vi "TH_Bladmögelvarning Skylt.vi"(7 "Tid":string) -> ()   [LabVIEW 2014]
panel:
  in  "OK Button":bool
  # "Bladmögelvarning !"
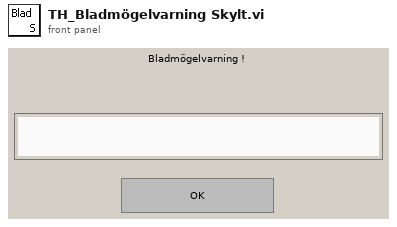
[diagram p1: front panel]
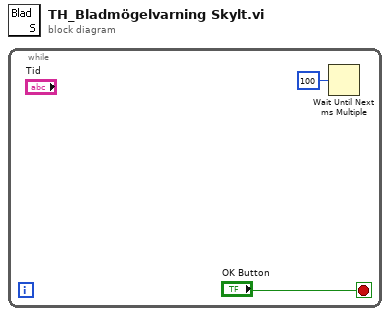
[diagram p0: block diagram]
diagram:
  n1 = while {
    stop <- "OK Button" stop-if-true
    n2 = Wait Until Next ms Multiple(millisecond multiple=u32 100) -> ()  [unwired: 1 out]
  }
